vi "controller connect.vi"(8 "IO on":bool, 9 "dispencer on":bool, 10 "motion on":bool, 11 "controller in":T1) -> (3 "controller out":T1)   [LabVIEW 2016]
uses:
  Classes/Controller/Motion/A3200 Folder/A3200.lvclass
  Classes/Controller/Dispenser/Ultimus V2 Folder/Ultimus V2.lvclass
  Classes/Controller/I-O/NI-DAQ Folder/NI-DAQ.lvclass
  Classes/Controller/Motion/Motion Folder/Motion.lvclass
  Classes/Controller/I-O/I-O Folder/I-O.lvclass
  Classes/Controller/Dispenser/Dispenser Folder/Dispenser.lvclass
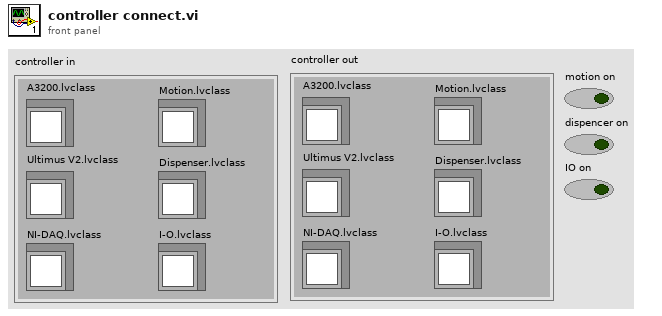
[diagram p1: front panel]
types:
  T1 = cluster{"A3200.lvclass":refnum<class "A3200.lvclass">, "Ultimus V2.lvclass":refnum<class "Ultimus V2.lvclass">, "NI-DAQ.lvclass":refnum<class "NI-DAQ.lvclass">, "Motion.lvclass":refnum<class "Motion.lvclass">, "I-O.lvclass":refnum<class "I-O.lvclass">, "Dispenser.lvclass":refnum<class "Dispenser.lvclass">}
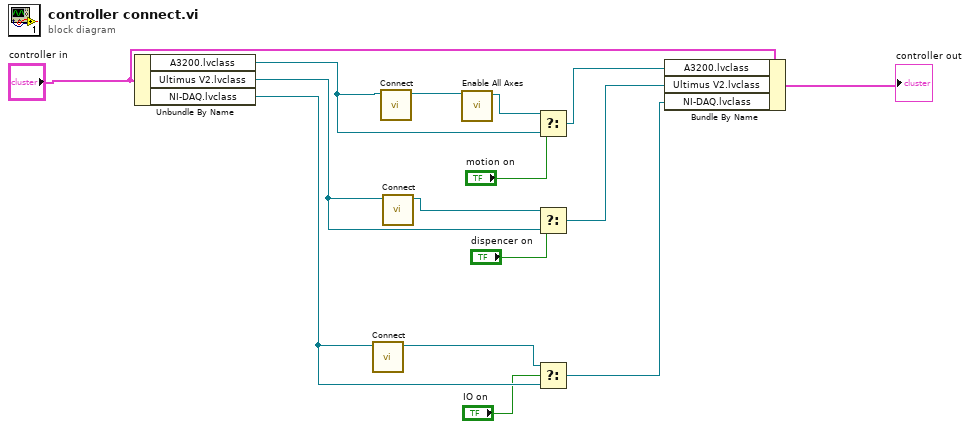
[diagram p0: block diagram]
diagram:
  n1 = Unbundle By Name("controller in") -> ("A3200.lvclass"=w15:refnum<class "A3200.lvclass">, "Ultimus V2.lvclass"=w7:refnum<class "Ultimus V2.lvclass">, "NI-DAQ.lvclass"=w12:refnum<class "NI-DAQ.lvclass">)
  n2 = call-dynamic "Connect.vi"("NI-DAQ in"=w12) -> ("NI-DAQ out"=w11:refnum<class "NI-DAQ.lvclass">)  [unwired: 9 in, 1 out]
  n3 = call-dynamic "Connect.vi"("Gantry in"=w15) -> ("Gantry out"=w14:refnum<class "A3200.lvclass">)  [unwired: 9 in, 1 out]
  n4 = call-dynamic "Connect.vi"("Ultimus V in"=w7) -> ("Ultimus V out"=w6:refnum<class "Ultimus V2.lvclass">)  [unwired: 9 in, 1 out]
  n5 = call-dynamic "Enable All Axes.vi"("A3200 in"=w14) -> ("A3200 out"=w13:refnum<class "A3200.lvclass">)  [unwired: 9 in, 1 out]
  n6 = Select(t=w13, s="motion on", f=w15) -> (s? t:f=w8:refnum<class "A3200.lvclass">)
  n7 = Select(t=w6, s="dispencer on", f=w7) -> (s? t:f=w9:refnum<class "Ultimus V2.lvclass">)
  n8 = Select(t=w11, s="IO on", f=w12) -> (s? t:f=w10:refnum<class "NI-DAQ.lvclass">)
  n9 = Bundle By Name(cluster="controller in", "A3200.lvclass"=w8, "Ultimus V2.lvclass"=w9, "NI-DAQ.lvclass"=w10) -> (→"controller out":T1)
